vi "U8arrayToMeasurement2.vi"(4 "payload":u8[](array[numeric]), 5 "factor 4":dbl=1000.0 format="%#_13g", 6 "factor 3":dbl=1000.0 format="%#_13g", 7 "factor 2":dbl=1000.0 format="%#_13g", 8 "factor 1":dbl=1000.0 format="%#_13g") -> (0 "Meas 4":dbl, 1 "Meas 3":dbl, 2 "Meas 2":dbl, 3 "uint16":u16)   [LabVIEW 2021]
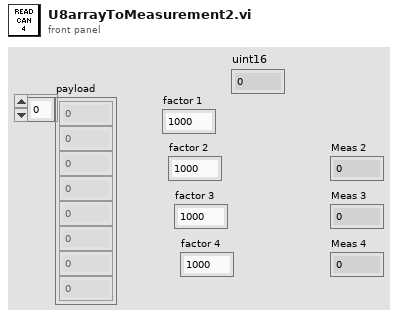
[diagram p1: front panel]
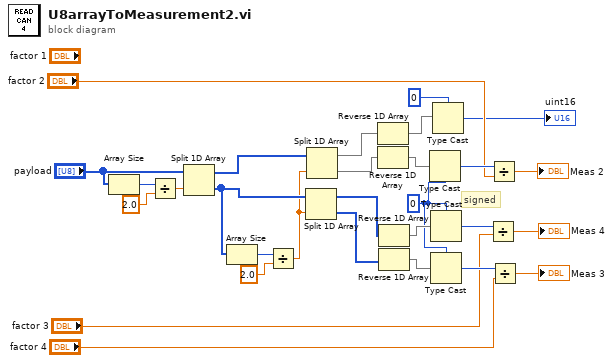
[diagram p0: block diagram]
diagram:
  w1 = i16 0
  # "signed"
  n1 = Array Size(array="payload") -> (size(s)=w26:i32)
  n2 = Divide(x=w26, y=2.0) -> (x/y=w28:dbl)
  n3 = Split 1D Array(array="payload", index=w28) -> (first subarray=w21:u8[], second subarray=w19:u8[])
  n4 = Array Size(array=w19) -> (size(s)=w6:i32)
  n5 = Divide(x=w6, y=2.0) -> (x/y=w18:dbl)
  n6 = Split 1D Array(array=w19, index=w18) -> (first subarray=w10:u8[], second subarray=w9:u8[])
  n7 = Split 1D Array(array=w21, index=w18) -> (first subarray=w17:u8[], second subarray=w5:u8[])
  n8 = Reverse 1D Array(array=w17) -> (reversed array=w4:u8[])
  n9 = Reverse 1D Array(array=w5) -> (reversed array=w29:u8[])
  n10 = Reverse 1D Array(array=w10) -> (reversed array=w14:u8[])
  n11 = Reverse 1D Array(array=w9) -> (reversed array=w15:u8[])
  n12 = Type Cast(type=w1, x=w29) -> (*(type *) &x=w24:i16)
  n13 = Type Cast(type=w1, x=w14) -> (*(type *) &x=w16:i16)
  n14 = Type Cast(type=w1, x=w15) -> (*(type *) &x=w13:i16)
  n15 = Type Cast(type=u16 0, x=w4) -> (*(type *) &x=→"uint16":u16)
  n16 = Divide(x=w16, y="factor 3") -> (x/y=→"Meas 4":dbl)
  n17 = Divide(x=w24, y="factor 2") -> (x/y=→"Meas 2":dbl)
  n18 = Divide(x=w13, y="factor 4") -> (x/y=→"Meas 3":dbl)
